vi "Add VIs to Library.vi"(8 "error in":errorcluster, 9 "Event Type":T1, 10 "Event VIs":refnum<vi>[](array[refnum]), 11 "Library In":refnum<class "Library.lvclass">) -> (0 "error out":errorcluster, 3 "Library Out":refnum<class "Library.lvclass">)   [LabVIEW 2019, in "Panther Dashboard.lvlib" / "Library.lvclass"]
uses:
  Library.lvclass
  VI/VI.lvclass
  VI/VI.lvclass/VI.ctl
  Library.lvclass/Library.ctl
  VI/Write VI Plain Name.vi
  VI/Write VI Path.vi
  Write VIs MAP.vi
  VI Type--enum.ctl
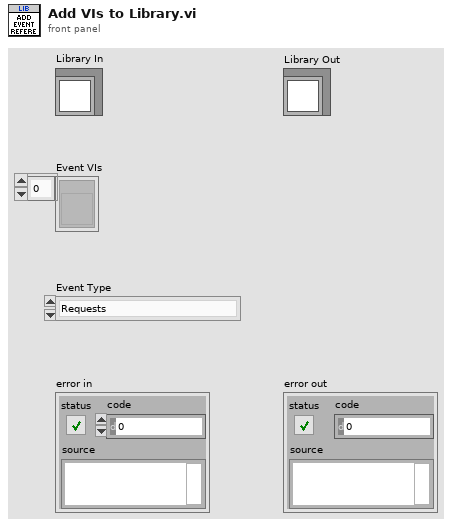
[diagram p1: front panel]
types:
  T1 = typedef "Panther Dashboard.lvlib/Library.lvclass/VI Type--enum.ctl" = enum16{"Requests", "Broadcasts", "Request and Wait for Reply", "Round Trips", "Public API VIs", "» Constant VIs", "» Error VIs"}
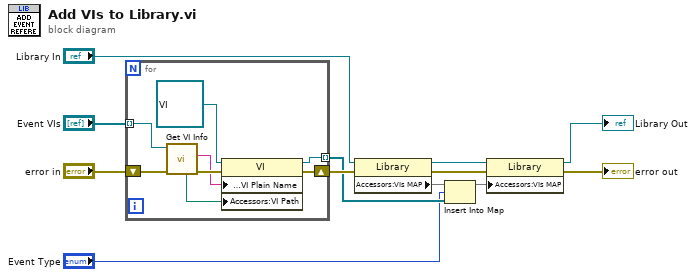
[diagram p0: block diagram]
diagram:
  n1 = for {
    tunnel: "Event VIs" -> [w17] mode=indexing
    tunnel: [w15] -> w2 mode=indexing
    shift-right: [w20] -> w11
    shift-left: "error in" -> [w19]
    n2 = call "Get VI Info.vi"("error in"=w19, "VI in"=w17) -> ("error out"=w18:errorcluster, "Plain Name"=w14:string, "VI Path"=w13:path)  [unwired: 5 in, 2 out]
    n3 = property class="VI"(reference=refnum<class "VI.lvclass"> refnum ("VI"), error in=w18, "Accessors:VI Plain Name"=w14, "Accessors:VI Path"=w13) -> (reference out=w15:refnum<class "VI.lvclass">, error out=w20:errorcluster)
  }
  n4 = property class="Library"(reference="Library In", error in=w11) -> (reference out=w5:refnum<class "Library.lvclass">, error out=w9:errorcluster, "Accessors:VIs MAP"=w4:map{T1, refnum<class "VI.lvclass">[]})
  n5 = Insert Into Map(map in=w4, key="Event Type", value=w2) -> (map out=w3:map{T1, refnum<class "VI.lvclass">[]})  [unwired: 2 out]
  n6 = property class="Library"(reference=w5, error in=w9, "Accessors:VIs MAP"=w3) -> (reference out=→"Library Out":refnum<class "Library.lvclass">, error out=→"error out":errorcluster)
